vi "filt2.vi"() -> ()   [LabVIEW 2010]
panel:
  in  "Enum":enum16{"rep", "square", "sin"}(ring)=enum."sin"
  in  "Noise amplitude":dbl
  out "size(s)":i32
  out "Array":dbl[](array[numeric])
  out "XY Graph":cluster{i32[], i16[]}[](graph)
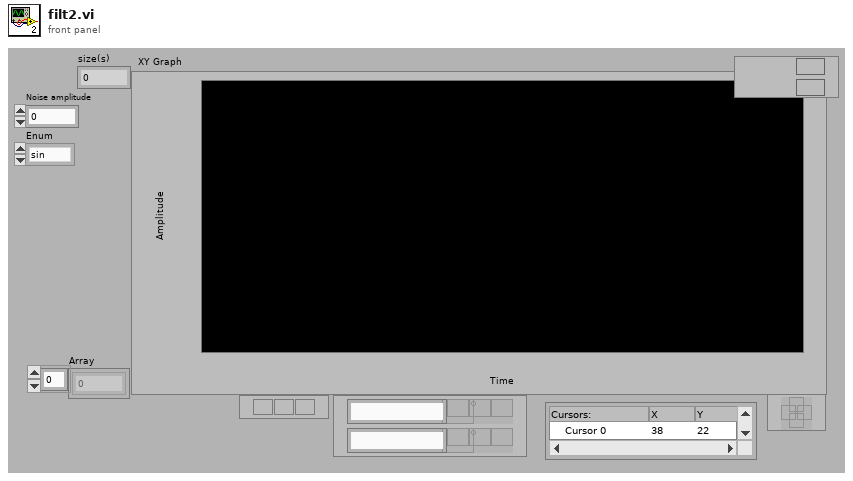
[diagram p1: front panel]
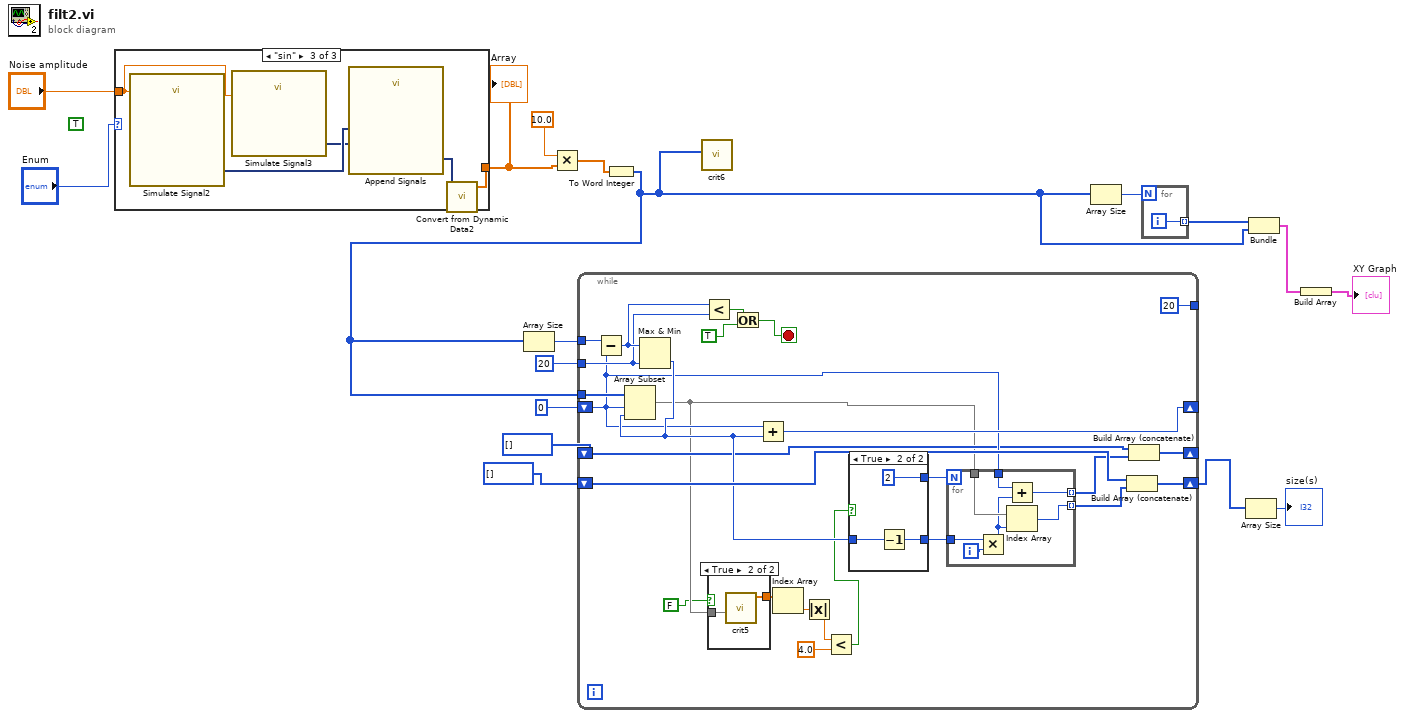
[diagram p0: block diagram]
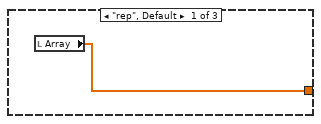
[diagram p2: hidden frame]
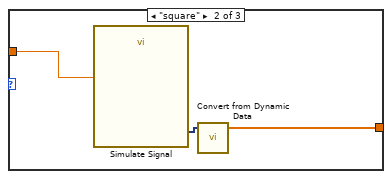
[diagram p3: hidden frame]
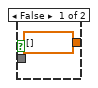
[diagram p4: hidden frame]
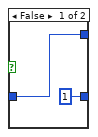
[diagram p5: hidden frame]
diagram:
  (unwired) TRUE
  n1 = case shown="\"sin\"" "Enum" {
    tunnel: [w18 w20 w26] -> w12
    tunnel: "Noise amplitude" -> [_ w19 w22]
    frame "rep", Default {
      n2 = local read "Array"() -> (w18:dbl[])
    }
    frame "square" {
      n3 = call "Simulate Signal"("Noise amplitude"=w19) -> ("Square with Uniform Noise"=w21:dynamicdata)  [unwired: 13 in, 1 out]
      n4 = call "Convert from Dynamic Data"("Dynamic Data Type"=w21) -> ("Array"=w20:dbl[])  [unwired: 3 in]
    }
    frame "sin" {
      n5 = call "Simulate Signal2"("Noise amplitude"=w22) -> ("Sine with Uniform Noise"=w25:dynamicdata)  [unwired: 13 in, 1 out]
      n6 = call "Simulate Signal3"("Noise amplitude"=w22) -> ("DC with Uniform Noise"=w24:dynamicdata)  [unwired: 13 in, 1 out]
      n7 = call "Append Signals"("Input Signal B"=w24, "Input Signal A"=w25) -> ("Appended Signals"=w23:dynamicdata)  [unwired: 8 in, 1 out]
      n8 = call "Convert from Dynamic Data2"("Dynamic Data Type"=w23) -> ("Array"=w26:dbl[])  [unwired: 3 in]
    }
  }
  "Array" <- w12
  n9 = Multiply(x=10.0 ("Noise amplitude"), y=w12) -> (x*y=w4:dbl[])
  n10 = To Word Integer(number=w4) -> (16bit integer=w1:i16[])
  n11 = Array Size(array=w1) -> (size(s)=w10:i32)
  n12 = while {
    shift-right: [w50] -> _
    shift-left: 0 -> [w38]
    tunnel: w1 -> [w51]
    tunnel: w10 -> [w49]
    tunnel: 20 -> [w47]
    shift-right: [w42] -> w6
    shift-left: i16[] [] ("subarray") -> [w43]
    shift-right: [w37] -> _
    shift-left: i32[] [] -> [w36]
    tunnel: [20 ("length")] -> _
    stop <- w45 stop-if-true
    n13 = Subtract(x=w49, y=w38) -> (x-y=w48:i32)
    n14 = Max & Min(x=w48, y=w47) -> (min(x,y)=w41:i32)  [unwired: 1 out]
    n15 = Array Subset(array=w51, index=w38, length=w41) -> (w34:i16[])
    n16 = Less?(x=w48, y=w47) -> (x < y?=w46:bool)
    n17 = case shown="True" FALSE {
      tunnel: w34 -> [_ w55]
      tunnel: [dbl[] [] ("C") w54] -> w33
      frame False {
      }
      frame True {
        n18 = call "crit5.vi"("ArrayIn"=w55) -> ("C"=w54:dbl[])  [unwired: 4 in, 2 out]
      }
    }
    n19 = Or(x=w46, y=TRUE) -> (x .or. y?=w45:bool)
    n20 = Add(x=w38, y=w41) -> (x+y=w50:i32)
    n21 = Index Array(array=w33) -> (element=w32:dbl)  [unwired: 1 in]
    n22 = Absolute Value(x=w32) -> (abs(x)=w29:dbl)
    n23 = Less?(x=w29, y=4.0) -> (x < y?=w30:bool)
    n24 = case shown="True" w30 {
      tunnel: w41 -> [w57 w60]
      tunnel: [1 w59] -> w40
      tunnel: [w57 2] -> w39
      frame False {
      }
      frame True {
        n25 = Decrement(x=w60) -> (x-1=w59:i32)
      }
    }
    n26 = for {
      N: w39 -> [_]
      tunnel: [w67] -> w44 mode=indexing
      tunnel: w34 -> [w66]
      tunnel: w40 -> [w64]
      tunnel: w38 -> [w63]
      tunnel: [w61] -> w35 mode=indexing
      i -> [w65]
      n27 = Multiply(x=w64, y=w65) -> (x*y=w62:i32)
      n28 = Add(x=w63, y=w62) -> (x+y=w61:i32)
      n29 = Index Array(array=w66, index=w62) -> (element=w67:i16)
    }
    n30 = Build Array (concatenate)(w43, w44) -> (w42:i16[])
    n31 = Build Array (concatenate)(w36, w35) -> (w37:i32[])
  }
  n32 = call "crit6.vi"("Array"=w1) -> ()  [unwired: 7 in]
  n33 = Array Size(array=w1) -> (size(s)=w16:i32)
  n34 = for {
    N: w16 -> [_]
    tunnel: [w68] -> w14 mode=indexing
    i -> [w68]
  }
  n35 = Array Size(array=w6) -> (size(s)=→"size(s)":i32)
  n36 = Bundle(w14, w1) -> (w15:cluster{i32[], i16[]})  [unwired: 1 in]
  n37 = Build Array(w15) -> (→"XY Graph":cluster{i32[], i16[]}[])
